vi "HEWH Special Last Draw Determine Purge Start.vi"(8 "Error In":errorcluster, 9 "Ideal Purge Time":dbl, 10 "Total Test Timer (1hr)":dbl, 11 "Current Draw Timer":dbl) -> (0 "Error Out":errorcluster, 2 "Start Purge":bool, 3 "Seconds Until EOT":dbl)   [LabVIEW 2016]
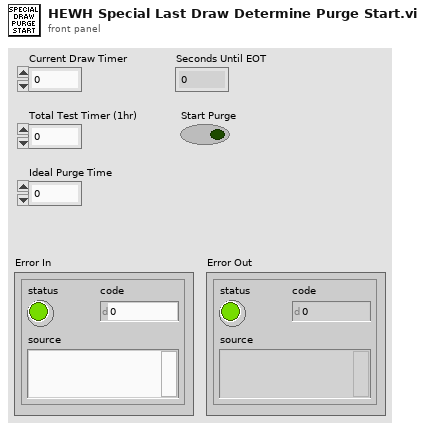
[diagram p1: front panel]
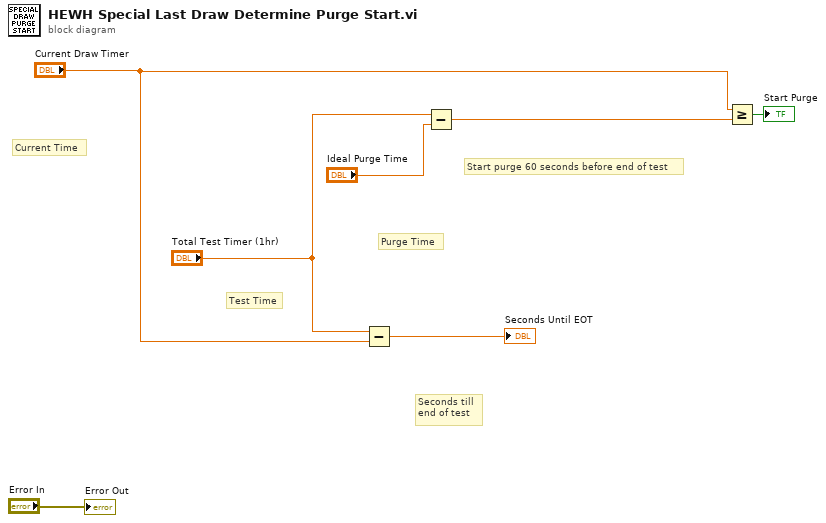
[diagram p0: block diagram]
diagram:
  # "Start purge 60 seconds before end of test"
  # "Seconds till \nend of test"
  # "Purge Time"
  # "Current Time"
  # "Test Time"
  n1 = Subtract(x="Total Test Timer (1hr)", y="Current Draw Timer") -> (x-y=→"Seconds Until EOT":dbl)
  n2 = Subtract(x="Total Test Timer (1hr)", y="Ideal Purge Time") -> (x-y=w2:dbl)
  n3 = Greater Or Equal?(x="Current Draw Timer", y=w2) -> (x >= y?=→"Start Purge":bool)
  "Error Out" <- "Error In"
